vi "Select State(s).vi"   [LabVIEW 2013]
doc: "Passes State(s) based on a condition\n\nFor instructions on how to use the JKI State Machine, examples and video tutorials, visit:\nhttp://jkisoft.com/state-machine/"
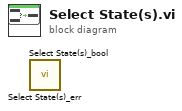
[diagram p0: block diagram]
diagram:
  n1 = call "Select State(s)_err.vi"() -> ()  [unwired: 15 in, 1 out]
  n2 = call "Select State(s)_bool.vi"() -> ()  [unwired: 15 in, 1 out]
